vi "LVClass_WavefrontCorrector Disconnect.vi"(0 "WavefrontCorrector in":refnum<class "WavefrontCorrector.lvclass">, 11 "error in (no error)":errorcluster) -> (4 "WavefrontCorrector out":refnum<class "WavefrontCorrector.lvclass">, 15 "error out":errorcluster)   [LabVIEW 2020, in "WavefrontCorrector.lvclass"]
doc: "Wavefront corrector parameter getter for parameter of type boolean.\n\n--------------------------------------------------------------------------------\n\n<B>correctorIn </B> : WavefrontCorrector object.\n<B>correctorOut </B> : WavefrontCorrector object.\n<B>parameter_name </B> : Name of the parameter.\n<B>value </B> : Value of the parameter.\n<B>ErrorIn </B> : Error\n<B>ErrorOut </B> : Error\n\n--------------------------------------------------------------------------------"
uses:
  WavefrontCorrector.lvclass
  WavefrontCorrector.lvclass/WavefrontCorrector.ctl
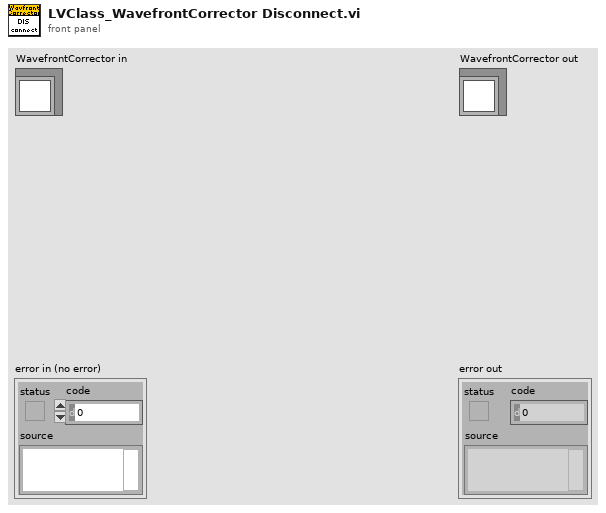
[diagram p1: front panel]
types:
  T1 = typedef "ClassID.ctl" = i64
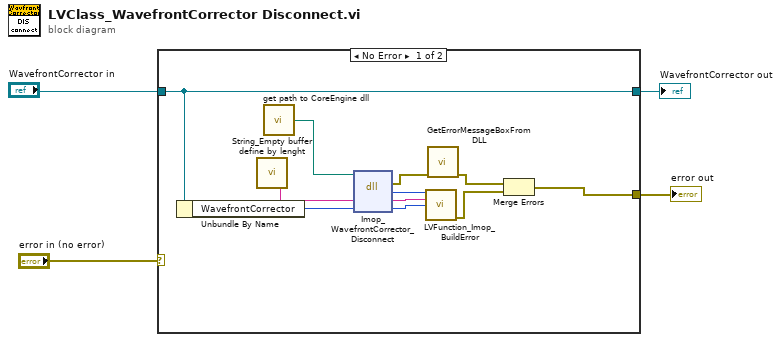
[diagram p0: block diagram]
diagram:
  n1 = case shown="No Error" "error in (no error)" {
    selector: "error in (no error)" -> [_ w17]
    tunnel: [w6 w17] -> w2
    tunnel: [w12 w16] -> w1
    tunnel: "WavefrontCorrector in" -> [w12 w16]
    frame No Error {
      n2 = Unbundle By Name(w12) -> ("WavefrontCorrector"=w13:T1)
      n3 = call "String_Empty buffer define by lenght.vi"() -> ("Empty buffer"=w9:string)  [unwired: 1 in]
      n4 = call "get path to CoreEngine dll.vi"() -> ("path to wavekit library"=w11:path)  [unwired: 14 in, 1 out]
      n5 = dll-call lib="D:/SOFTware/CoreEngine4_Suite/SVN_trunk/LV2011_interface/DLLs/c_interface_vc100.dll" fn="Imop_WavefrontCorrector_Disconnect"(path in=w11, "message"=w9, "camera"=w13) -> (error out=w10:errorcluster, "return type"=w15:i32, "message"=w14:string, "camera"=w5:i64)  [unwired: 2 in, 1 out]
      n6 = call "LVFunction_Imop_BuildError.vi"("code"=w15, "String to Prepend to source (\"\")"=w14, "Adresse"=w5) -> ("error out"=w7:errorcluster)  [unwired: 12 in]
      n7 = call "GetErrorMessageBoxFromDLL.vi"("error IN"=w10) -> ("error OUT"=w8:errorcluster)  [unwired: 10 in]
      n8 = Merge Errors(w8, w7) -> (w6:errorcluster)
    }
    frame Error {
    }
  }
  "error out" <- w2
  "WavefrontCorrector out" <- w1
